vi "Update Mode.vi"(9 "Options":u16(ring) items=["volts DC", "volts AC", "2-wire k.ohms", "4-wire k.ohms", "mA DC", "mA AC"], 11 "multimeter in":refnum<class "Fluke Multimeter.lvclass">) -> (3 "multimeter out":refnum<class "Fluke Multimeter.lvclass">)   [LabVIEW 2012, in "Fluke Multimeter.lvclass"]
uses:
  Fluke Multimeter.lvclass
  Fluke Multimeter.lvclass/Fluke Multimeter.ctl
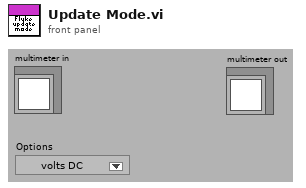
[diagram p1: front panel]
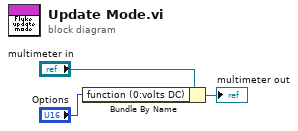
[diagram p0: block diagram]
diagram:
  n1 = Bundle By Name(cluster="multimeter in", "function (0:volts DC)"="Options") -> (→"multimeter out":refnum<class "Fluke Multimeter.lvclass">)
